vi "WSVCAP SHL Host LL I2C Convert Channel Bytes to Bit Array.vi"(0 "C1 Data Out":u8[][](array[numeric]) format="%.0x", 5 "C2 Data Out":u8[][](array[numeric]) format="%.0x", 7 "C3 Data Out":u8[][](array[numeric]) format="%.0x") -> (4 "Write Data":u64[](array[numeric]) format="%032b")   [LabVIEW 2012]
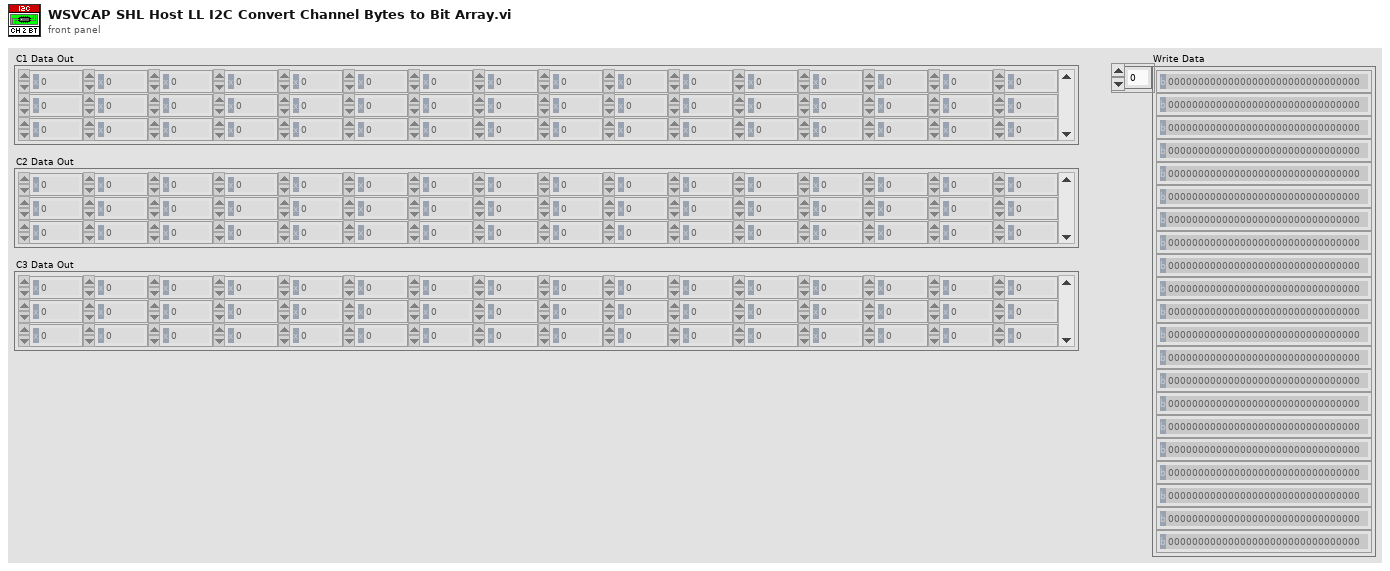
[diagram p1: front panel]
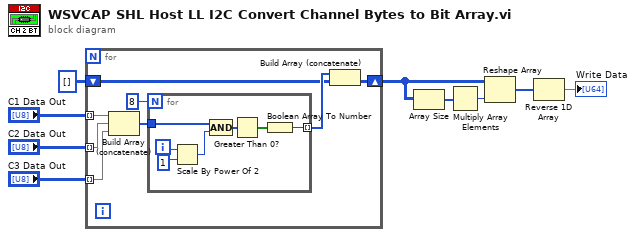
[diagram p0: block diagram]
diagram:
  n1 = for {
    tunnel: "C1 Data Out" -> [w17] mode=indexing
    tunnel: "C2 Data Out" -> [w16] mode=indexing
    shift-right: [w12] -> w2
    shift-left: u64[][] [] -> [w11]
    tunnel: "C3 Data Out" -> [w10] mode=indexing
    n2 = Build Array (concatenate)(w17, w16, w10) -> (w15:u8[])
    n3 = for {
      N: 8 -> [_]
      tunnel: w15 -> [w20]
      tunnel: [w19] -> w13 mode=indexing
      i -> [w22]
      n4 = Scale By Power Of 2(n=w22, x=u8 1) -> (x*2^n=w23:u8)
      n5 = Compound Arithmetic op=AND(w20, w23) -> (w24:u8[])
      n6 = Greater Than 0?(x=w24) -> (x > 0?=w18:bool[])
      n7 = Boolean Array To Number(Boolean array=w18) -> (number=w19:u64)
    }
    n8 = Build Array (concatenate)(w13, w11) -> (w12:u64[][])
  }
  n9 = Array Size(array=w2) -> (size(s)=w7:i32[])
  n10 = Multiply Array Elements(1:w7) -> (0:w6:i32)
  n11 = Reshape Array(w2, w6) -> (w5:u64[])
  n12 = Reverse 1D Array(array=w5) -> (reversed array=→"Write Data":u64[])
